vi "Node - Type Cast.vi"(8 "error in (no error)":errorcluster, 10 "Node Local Channels":T1[](array[typedef]), 11 "Byte Buffer In":refnum<class "Byte Buffer.lvclass">) -> (0 "error out":errorcluster, 2 "Buffer Offset Out":u64, 3 "Byte Buffer Out":refnum<class "Byte Buffer.lvclass">)   [LabVIEW 2016, in "PXImc Router.lvlib"]
uses:
  PXImc Router.lvlib
  Controls/Node/Node Ch Properties.ctl
  Controls/Data Type.ctl
  <vilib>/NI Veristand/VeriStand Data/Byte Buffer/Byte Buffer.lvclass
  <vilib>/NI Veristand/VeriStand Data/Byte Buffer/Byte Buffer.lvclass/Byte Buffer.ctl
  <vilib>/NI Veristand/VeriStand Data/Byte Buffer/Byte Buffer.Write (Boolean).vi
  <vilib>/NI Veristand/VeriStand Data/Type Conversion/Type Conversion.From Double (Boolean).vi
  <vilib>/NI Veristand/VeriStand Data/Byte Buffer/Byte Buffer.Write (SGL).vi
  <vilib>/NI Veristand/VeriStand Data/Type Conversion/Type Conversion.From Double (SGL).vi
  <vilib>/NI Veristand/VeriStand Data/Byte Buffer/Byte Buffer.Write (DBL).vi
  <vilib>/NI Veristand/VeriStand Data/Byte Buffer/Byte Buffer.Write (I8).vi
  <vilib>/NI Veristand/VeriStand Data/Type Conversion/Type Conversion.From Double (I8).vi
  <vilib>/NI Veristand/VeriStand Data/Byte Buffer/Byte Buffer.Write (I16).vi
  <vilib>/NI Veristand/VeriStand Data/Type Conversion/Type Conversion.From Double (I16).vi
  <vilib>/NI Veristand/VeriStand Data/Byte Buffer/Byte Buffer.Write (I32).vi
  <vilib>/NI Veristand/VeriStand Data/Type Conversion/Type Conversion.From Double (I32).vi
  <vilib>/NI Veristand/VeriStand Data/Byte Buffer/Byte Buffer.Write (I64).vi
  <vilib>/NI Veristand/VeriStand Data/Type Conversion/Type Conversion.From Double (I64).vi
  <vilib>/NI Veristand/VeriStand Data/Byte Buffer/Byte Buffer.Write (U8).vi
  <vilib>/NI Veristand/VeriStand Data/Type Conversion/Type Conversion.From Double (U8).vi
  <vilib>/NI Veristand/VeriStand Data/Byte Buffer/Byte Buffer.Write (U16).vi
  <vilib>/NI Veristand/VeriStand Data/Type Conversion/Type Conversion.From Double (U16).vi
  <vilib>/NI Veristand/VeriStand Data/Byte Buffer/Byte Buffer.Write (U32).vi
  <vilib>/NI Veristand/VeriStand Data/Type Conversion/Type Conversion.From Double (U32).vi
  <vilib>/NI Veristand/VeriStand Data/Byte Buffer/Byte Buffer.Write (U64).vi
  <vilib>/NI Veristand/VeriStand Data/Type Conversion/Type Conversion.From Double (U64).vi
  <vilib>/NI Veristand/VeriStand Data/Byte Buffer/Byte Buffer.Write (String).vi
  <vilib>/NI Veristand/VeriStand Data/Byte Buffer/Byte Buffer.Subset.Set.vi
  <vilib>/NI Veristand/VeriStand Data/Byte Buffer/Byte Buffer.Get Buffer Pointer.vi
  <vilib>/NI Veristand/VeriStand Data/Byte Buffer/Byte Buffer.Get Buffer Size.vi
  <vilib>/NI Veristand/VeriStand Data/Memory Management/Memory Management.MoveByteBlock.Read (String).vi
  <vilib>/NI Veristand/VeriStand Data/Memory Management/Memory Management.Handle Return.vi
  <vilib>/NI Veristand/VeriStand Data/Byte Buffer/Byte Buffer.Get Byte Order.vi
  <vilib>/NI Veristand/VeriStand Data/VeriStand Data.lvlib
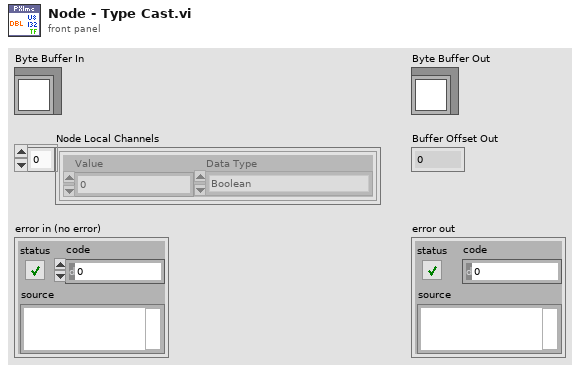
[diagram p1: front panel]
types:
  T1 = typedef "PXImc Router.lvlib/Node Ch Properties.ctl" = cluster{"Value":dbl, "Data Type":T2}
  T2 = typedef "PXImc Router.lvlib/Data Type.ctl" = enum16{"Boolean", "SGL", "DBL", "I8", "I16", "I32", "I64", "U8", "U16", "U32", "U64"}
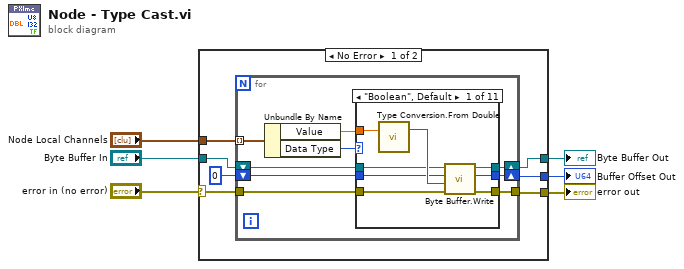
[diagram p0: block diagram]
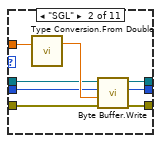
[diagram p2: hidden frame]
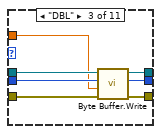
[diagram p3: hidden frame]
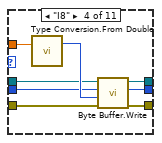
[diagram p4: hidden frame]
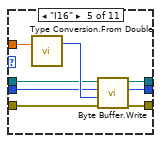
[diagram p5: hidden frame]
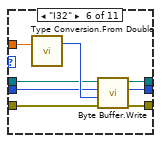
[diagram p6: hidden frame]
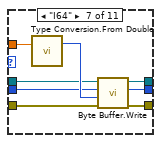
[diagram p7: hidden frame]
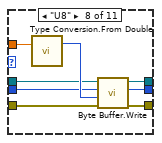
[diagram p8: hidden frame]
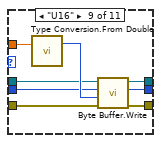
[diagram p9: hidden frame]
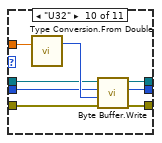
[diagram p10: hidden frame]
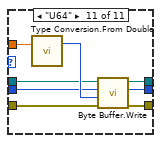
[diagram p11: hidden frame]
diagram:
  n1 = case shown="No Error" "error in (no error)" {
    selector: "error in (no error)" -> [w7 w110]
    tunnel: "Node Local Channels" -> [w13 _]
    tunnel: [w12 _] -> w5
    tunnel: [w11 w110] -> w4
    tunnel: [w10 w111] -> w3
    tunnel: "Byte Buffer In" -> [w8 w111]
    frame No Error {
      n2 = for {
        tunnel: [w21] -> w11
        shift-right: [w22] -> w10
        shift-left: w8 -> [w20]
        shift-right: [w19] -> w12
        shift-left: u64 0 ("new buffer offset") -> [w18]
        tunnel: w7 -> [w17]
        tunnel: w13 -> [w16] mode=indexing
        n3 = Unbundle By Name(w16) -> ("Value"=w14:dbl, "Data Type"=w15:T2)
        n4 = case shown="\"Boolean\", Default" w15 {
          tunnel: [w29 w37 w45 w52 w60 w68 w76 w84 w92 w100 w108] -> w22
          tunnel: [w28 w36 w44 w51 w59 w67 w75 w83 w91 w99 w107] -> w21
          tunnel: w14 -> [w27 w35 w39 w50 w58 w66 w74 w82 w90 w98 w106]
          tunnel: w20 -> [w26 w34 w43 w49 w57 w65 w73 w81 w89 w97 w105]
          tunnel: [w25 w33 w42 w48 w56 w64 w72 w80 w88 w96 w104] -> w19
          tunnel: w18 -> [w23 w32 w41 w47 w55 w63 w71 w79 w87 w95 w103]
          tunnel: w17 -> [w24 w31 w40 w46 w54 w62 w70 w78 w86 w94 w102]
          frame "Boolean", Default {
            n5 = call-poly <vilib>:"Type Conversion.From Double.vi"("value in"=w27) -> ("value out"=w30:bool)  [unwired: 2 in]
            n6 = call-poly <vilib>:"Byte Buffer.Write.vi"("error in (no error)"=w24, "value"=w30, "buffer offset"=w23, "Byte Buffer in"=w26) -> ("error out"=w28:errorcluster, "new buffer offset"=w25:u64, "Byte Buffer out"=w29:refnum<class "Byte Buffer.lvclass">)  [unwired: 5 in]
          }
          frame "SGL" {
            n7 = call-poly <vilib>:"Type Conversion.From Double.vi"("value in"=w35) -> ("value out"=w38:sgl)  [unwired: 2 in]
            n8 = call-poly <vilib>:"Byte Buffer.Write.vi"("error in (no error)"=w31, "value"=w38, "buffer offset"=w32, "Byte Buffer in"=w34) -> ("error out"=w36:errorcluster, "new buffer offset"=w33:u64, "Byte Buffer out"=w37:refnum<class "Byte Buffer.lvclass">)  [unwired: 5 in]
          }
          frame "DBL" {
            n9 = call-poly <vilib>:"Byte Buffer.Write.vi"("error in (no error)"=w40, "value"=w39, "buffer offset"=w41, "Byte Buffer in"=w43) -> ("error out"=w44:errorcluster, "new buffer offset"=w42:u64, "Byte Buffer out"=w45:refnum<class "Byte Buffer.lvclass">)  [unwired: 5 in]
          }
          frame "I8" {
            n10 = call-poly <vilib>:"Type Conversion.From Double.vi"("value in"=w50) -> ("value out"=w53:i8)  [unwired: 2 in]
            n11 = call-poly <vilib>:"Byte Buffer.Write.vi"("error in (no error)"=w46, "value"=w53, "buffer offset"=w47, "Byte Buffer in"=w49) -> ("error out"=w51:errorcluster, "new buffer offset"=w48:u64, "Byte Buffer out"=w52:refnum<class "Byte Buffer.lvclass">)  [unwired: 5 in]
          }
          frame "I16" {
            n12 = call-poly <vilib>:"Type Conversion.From Double.vi"("value in"=w58) -> ("value out"=w61:i16)  [unwired: 2 in]
            n13 = call-poly <vilib>:"Byte Buffer.Write.vi"("error in (no error)"=w54, "value"=w61, "buffer offset"=w55, "Byte Buffer in"=w57) -> ("error out"=w59:errorcluster, "new buffer offset"=w56:u64, "Byte Buffer out"=w60:refnum<class "Byte Buffer.lvclass">)  [unwired: 5 in]
          }
          frame "I32" {
            n14 = call-poly <vilib>:"Type Conversion.From Double.vi"("value in"=w66) -> ("value out"=w69:i32)  [unwired: 2 in]
            n15 = call-poly <vilib>:"Byte Buffer.Write.vi"("error in (no error)"=w62, "value"=w69, "buffer offset"=w63, "Byte Buffer in"=w65) -> ("error out"=w67:errorcluster, "new buffer offset"=w64:u64, "Byte Buffer out"=w68:refnum<class "Byte Buffer.lvclass">)  [unwired: 5 in]
          }
          frame "I64" {
            n16 = call-poly <vilib>:"Type Conversion.From Double.vi"("value in"=w74) -> ("value out"=w77:i64)  [unwired: 2 in]
            n17 = call-poly <vilib>:"Byte Buffer.Write.vi"("error in (no error)"=w70, "value"=w77, "buffer offset"=w71, "Byte Buffer in"=w73) -> ("error out"=w75:errorcluster, "new buffer offset"=w72:u64, "Byte Buffer out"=w76:refnum<class "Byte Buffer.lvclass">)  [unwired: 5 in]
          }
          frame "U8" {
            n18 = call-poly <vilib>:"Type Conversion.From Double.vi"("value in"=w82) -> ("value out"=w85:u8)  [unwired: 2 in]
            n19 = call-poly <vilib>:"Byte Buffer.Write.vi"("error in (no error)"=w78, "value"=w85, "buffer offset"=w79, "Byte Buffer in"=w81) -> ("error out"=w83:errorcluster, "new buffer offset"=w80:u64, "Byte Buffer out"=w84:refnum<class "Byte Buffer.lvclass">)  [unwired: 5 in]
          }
          frame "U16" {
            n20 = call-poly <vilib>:"Type Conversion.From Double.vi"("value in"=w90) -> ("value out"=w93:u16)  [unwired: 2 in]
            n21 = call-poly <vilib>:"Byte Buffer.Write.vi"("error in (no error)"=w86, "value"=w93, "buffer offset"=w87, "Byte Buffer in"=w89) -> ("error out"=w91:errorcluster, "new buffer offset"=w88:u64, "Byte Buffer out"=w92:refnum<class "Byte Buffer.lvclass">)  [unwired: 5 in]
          }
          frame "U32" {
            n22 = call-poly <vilib>:"Type Conversion.From Double.vi"("value in"=w98) -> ("value out"=w101:u32)  [unwired: 2 in]
            n23 = call-poly <vilib>:"Byte Buffer.Write.vi"("error in (no error)"=w94, "value"=w101, "buffer offset"=w95, "Byte Buffer in"=w97) -> ("error out"=w99:errorcluster, "new buffer offset"=w96:u64, "Byte Buffer out"=w100:refnum<class "Byte Buffer.lvclass">)  [unwired: 5 in]
          }
          frame "U64" {
            n24 = call-poly <vilib>:"Type Conversion.From Double.vi"("value in"=w106) -> ("value out"=w109:u64)  [unwired: 2 in]
            n25 = call-poly <vilib>:"Byte Buffer.Write.vi"("error in (no error)"=w102, "value"=w109, "buffer offset"=w103, "Byte Buffer in"=w105) -> ("error out"=w107:errorcluster, "new buffer offset"=w104:u64, "Byte Buffer out"=w108:refnum<class "Byte Buffer.lvclass">)  [unwired: 5 in]
          }
        }
      }
    }
    frame Error {
    }
  }
  "Buffer Offset Out" <- w5
  "error out" <- w4
  "Byte Buffer Out" <- w3
